vi "OpenCVCam_SendUiEvent.vi"(7 "UiEventNames":T1, 8 "ErrorIn":errorcluster, 9 "Data":variant, 11 "OpenCVCamIn":refnum<class "OpenCVCam.lvclass">) -> (0 "ErrorOut":errorcluster, 3 "OpenCVCamOut":refnum<class "OpenCVCam.lvclass">)   [LabVIEW 2021, in "OpenCVCam.lvclass"]
uses:
  OpenCVCam.lvclass
  OpenCVCam_UiCallBackEvents.ctl
  OpenCVCam.lvclass/OpenCVCam.ctl
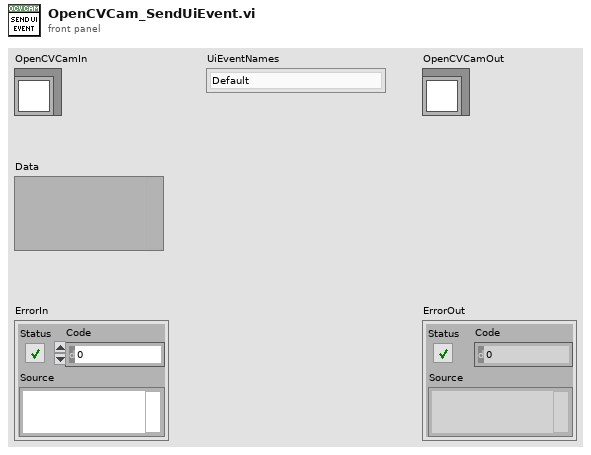
[diagram p1: front panel]
types:
  T1 = typedef "OpenCVCam.lvclass/OpenCVCam_UiCallBackEvents.ctl" = enum16{"Default", "PersistentDataUpdated", "NewPicture", "Worker 1: Do Something"}
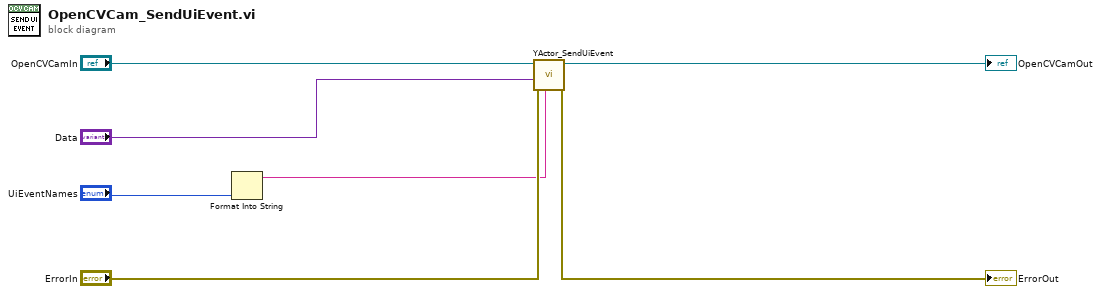
[diagram p0: block diagram]
diagram:
  n1 = Format Into String("UiEventNames") -> (resulting string=w2:string)  [unwired: 3 in, 1 out]
  n2 = call-dynamic "YActor_SendUiEvent.vi"("Event"=w2, "ErrorIn"="ErrorIn", "Data"="Data", "YActorIn"="OpenCVCamIn") -> ("ErrorOut"=→"ErrorOut":errorcluster, "YActorOut"=→"OpenCVCamOut":refnum<class "OpenCVCam.lvclass">)  [unwired: 6 in]
